vi "Read with timeout test.vi"() -> ()   [LabVIEW 2015]
uses:
  Controls/Sample Transfer Control Enumerator.ctl
panel:
  out "Numeric":i32
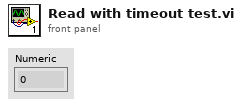
[diagram p1: front panel]
types:
  T1 = typedef "Sample Transfer Control Enumerator.ctl" = enum16{"Acknowledged", "Transfer", "Stash", "Abort", "Reset to Idle"}
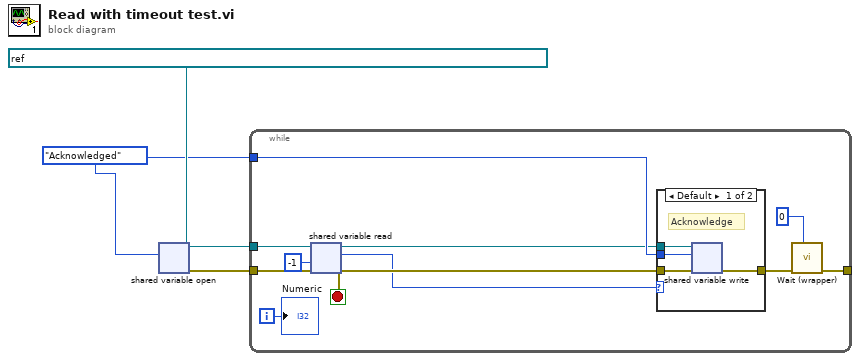
[diagram p0: block diagram]
diagram:
  w2 = Sample_Transfer_Control_Enumerator."Acknowledged" ("Sample Transfer Control")
  n1 = shared-variable-open(refnum<k21> "ni.var.psp://crio-carbondioxide/AMS Gas SHV/Sample Transfer/Control" ("shared variable refnum in"), w2) -> (w1:refnum<k21>, w4:errorcluster)  [unwired: 2 in]
  n2 = while {
    tunnel: w2 -> [w12]
    tunnel: [w13] -> _
    tunnel: w4 -> [w9]
    tunnel: w1 -> [w8]
    i -> [w7]
    stop <- w11 stop-if-true
    n3 = shared-variable-read(w8, w9, -1 ("timeout ms")) -> (w10:refnum<k21>, w11:errorcluster, w5:T1)  [unwired: 2 out]
    n4 = case shown="Default" w5 {
      tunnel: w10 -> [w19 _]
      tunnel: w11 -> [w18 w20]
      tunnel: w12 -> [w17 _]
      tunnel: [w16 w20] -> w14
      frame Default {
        # "Acknowledge"
        n5 = shared-variable-write(w19, w18, w17) -> (w16:errorcluster)  [unwired: 1 out]
      }
      frame "Acknowledged" {
      }
    }
    n6 = call "Wait (wrapper).vi"("milliseconds to wait (200)"=u32 0, "error in (no error)"=w14) -> ("error out"=w13:errorcluster)  [unwired: 9 in]
    "Numeric" <- w7
  }
